vi "split_pixels.vi"(8 "error in (no error)":errorcluster, 10 "pixels in":dbl[](array[numeric]), 11 "DL090211FrameImageAssembler in":refnum<class "ImageAssemblerDL090211Frame.lvclass">) -> (0 "error out":errorcluster, 1 "pixel block":sgl[][](array[numeric]), 2 "for next time":dbl[](array[numeric]), 3 "DL090211FrameImageAssembler out":refnum<class "ImageAssemblerDL090211Frame.lvclass">, 4 "end of frame reached?":bool, 5 "insertion coordinate":T1, 6 "another insertion possible?":bool, 7 "next inseration coordinate":u64)   [LabVIEW 2010, in "ImageAssemblerDL090211Frame.lvclass"]
uses:
  ImageAssemblerDL090211Frame.lvclass
  common/clusters/pixel_coordinate_cluster.ctl
  ImageAssemblerDL090211Frame.lvclass/ImageAssemblerDL090211Frame.ctl
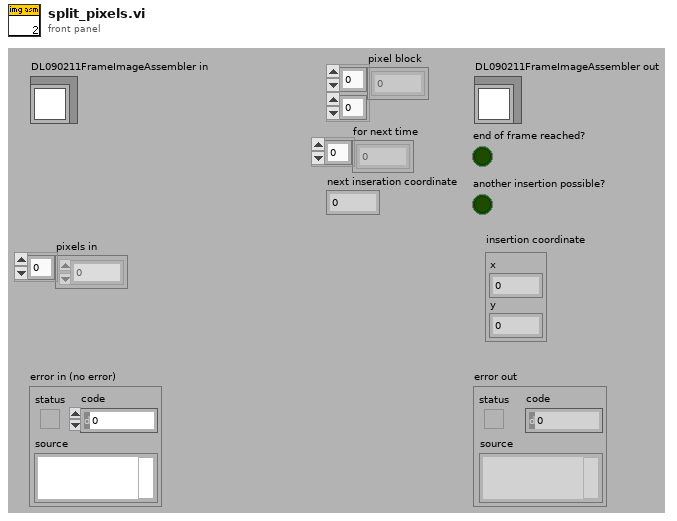
[diagram p1: front panel]
types:
  T1 = typedef "pixel_coordinate_cluster.ctl" = cluster{"x":i32, "y":i32}
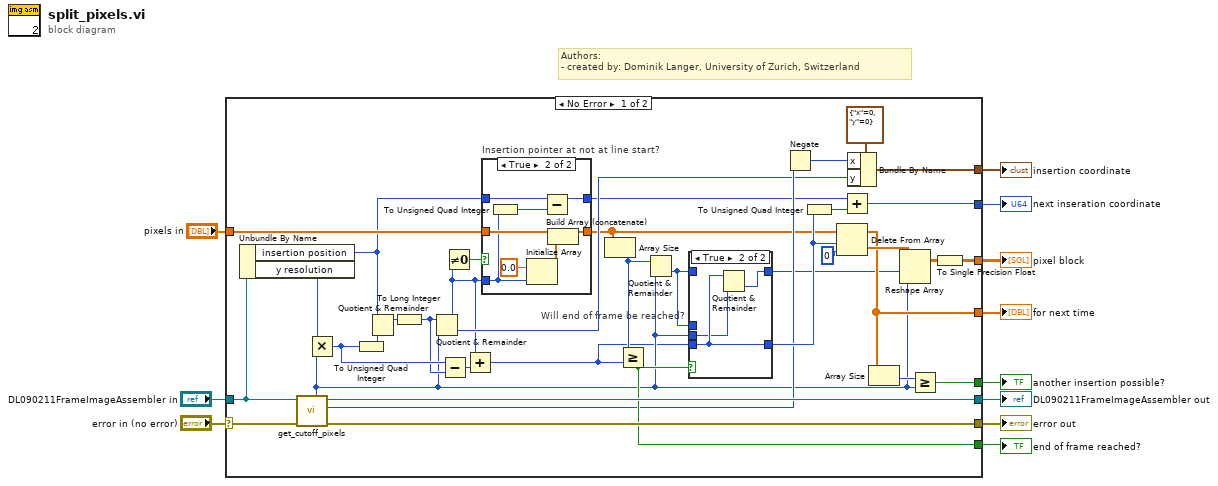
[diagram p0: block diagram]
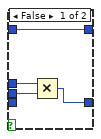
[diagram p3: hidden frame]
diagram:
  # "Authors: \n- created by: Dominik Langer, University of Zurich, Switzerland"
  n1 = case shown="No Error" "error in (no error)" {
    selector: "error in (no error)" -> [w48 w67]
    tunnel: [w43 w67] -> w10
    tunnel: [w42 w66] -> w8
    tunnel: "DL090211FrameImageAssembler in" -> [w46 w66]
    tunnel: [w37 _] -> w7
    tunnel: [w47 _] -> w6
    tunnel: [w28 _] -> w5
    tunnel: [w44 _] -> w4
    tunnel: "pixels in" -> [w21 _]
    tunnel: [w35 _] -> w2
    tunnel: [w32 _] -> w1
    frame No Error {
      n2 = Unbundle By Name(w46) -> ("insertion position"=w19:u64, "y resolution"=w30:i32)
      n3 = call-dynamic "get_cutoff_pixels.vi"("error in (no error)"=w48, "DL090211FrameImageAssembler in"=w46) -> ("error out"=w43:errorcluster, "left cut-off"=w27:i32, "DL090211FrameImageAssembler out"=w42:refnum<class "ImageAssemblerDL090211Frame.lvclass">, "total pixels per line"=w24:i32)  [unwired: 6 out]
      n4 = Multiply(x=w30, y=w24) -> (x*y=w39:i32)
      n5 = To Unsigned Quad Integer(1:w39) -> (0:w41:u64)
      n6 = Quotient & Remainder(x=w19, y=w41) -> (x-y*floor(x/y)=w40:u64)  [unwired: 1 out]
      n7 = To Long Integer(number=w40) -> (32bit integer=w31:i32)
      n8 = Quotient & Remainder(x=w31, y=w24) -> (x-y*floor(x/y)=w15:i32, floor(x/y)=w23:i32)
      n9 = Subtract(x=w39, y=w31) -> (x-y=w16:i32)
      n10 = Not Equal To 0?(x=w15) -> (x != 0?=w22:bool)
      n11 = Add(x=w15, y=w16) -> (x+y=w17:i32)
      n12 = case "Insertion pointer at not at line start?" shown="True" w22 {
        tunnel: w15 -> [_ w51]
        tunnel: w21 -> [w50 w57]
        tunnel: [w50 w55] -> w20
        tunnel: w19 -> [w49 w54]
        tunnel: [w49 w53] -> w18
        frame False {
        }
        frame True {
          n13 = To Unsigned Quad Integer(1:w51) -> (0:w52:u64)
          n14 = Initialize Array(0.0 ("element"), w51) -> (w56:dbl[])
          n15 = Subtract(x=w54, y=w52) -> (x-y=w53:u64)
          n16 = Build Array (concatenate)(w57, w56) -> (w55:dbl[])
        }
      }
      n17 = Array Size(array=w20) -> (size(s)=w38:i32)
      n18 = Greater Or Equal?(x=w38, y=w17) -> (x >= y?=w37:bool)
      n19 = Quotient & Remainder(x=w38, y=w24) -> (floor(x/y)=w13:i32)  [unwired: 1 out]
      n20 = case "Will end of frame be reached?" shown="True" w37 {
        tunnel: w17 -> [_ w65]
        tunnel: [w60 w65] -> w34
        tunnel: w13 -> [w61 _]
        tunnel: w24 -> [w62 w64]
        tunnel: w13 -> [w59 _]
        tunnel: [w59 w63] -> w12
        frame False {
          n21 = Multiply(x=w61, y=w62) -> (x*y=w60:i32)
        }
        frame True {
          n22 = Quotient & Remainder(x=w65, y=w64) -> (floor(x/y)=w63:i32)  [unwired: 1 out]
        }
      }
      n23 = Negate(x=w27) -> (-x=w26:i32)
      n24 = To Unsigned Quad Integer(1:w34) -> (0:w36:u64)
      n25 = Delete From Array(array=w20, length=w34, index=0) -> (deleted portion=w29:dbl[], array with subset deleted=w28:dbl[])
      n26 = Add(x=w18, y=w36) -> (x+y=w35:u64)
      n27 = Bundle By Name(cluster=T1 {"x"=0, "y"=0} ("next insertion coordinate"), "x"=w26, "y"=w23) -> (w32:T1)
      n28 = Array Size(array=w28) -> (size(s)=w45:i32)
      n29 = Reshape Array(w29, w12, w24) -> (w25:dbl[][])
      n30 = Greater Or Equal?(x=w45, y=w24) -> (x >= y?=w44:bool)
      n31 = To Single Precision Float(number=w25) -> (single precision float=w47:sgl[][])
    }
    frame Error {
    }
  }
  "error out" <- w10
  "DL090211FrameImageAssembler out" <- w8
  "insertion coordinate" <- w1
  "end of frame reached?" <- w7
  "pixel block" <- w6
  "for next time" <- w5
  "another insertion possible?" <- w4
  "next inseration coordinate" <- w2
